vi "DAB Encode.vi"(10 "Message":string, 11 "image data":T1) -> (3 "Encoded Image":T1)   [LabVIEW 2020]
uses:
  <vilib>/picture/picture.llb/imagedata.ctl
panel:
  out "Encoded Bytes":i32
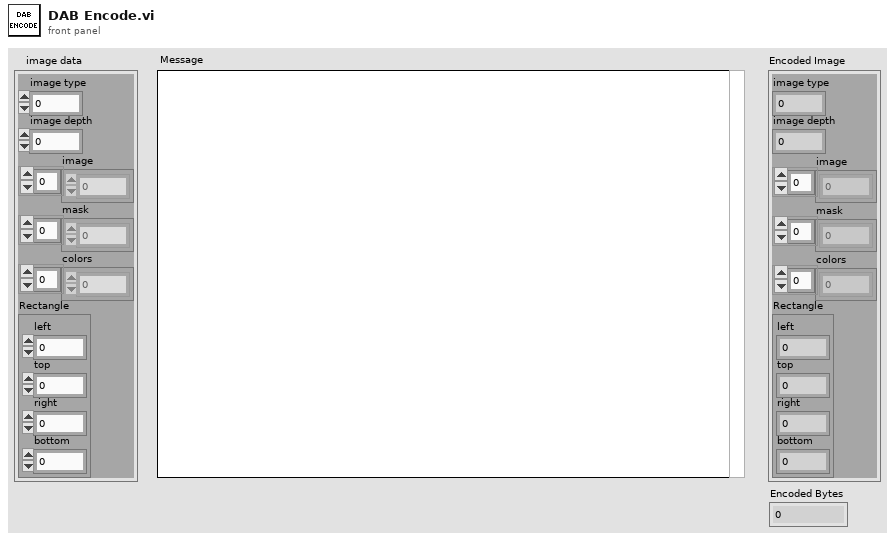
[diagram p1: front panel]
types:
  T1 = typedef "imagedata.ctl" = cluster{"image type":i32, "image depth":i32, "image":u8[], "mask":u8[], "colors":u32[], "Rectangle":cluster{"left":i16, "top":i16, "right":i16, "bottom":i16}}
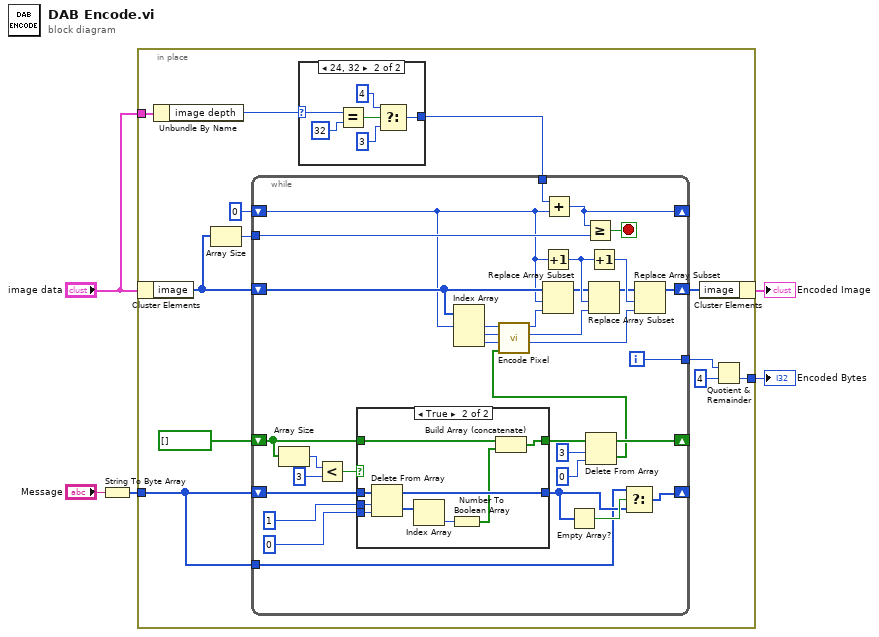
[diagram p0: block diagram]
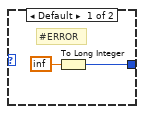
[diagram p3: hidden frame]
diagram:
  n1 = String To Byte Array(string="Message") -> (unsigned byte array=w2:u8[])
  n2 = in-place {
    in-place-border: "image data" -> [w17]
    in-place-border: w2 -> [w9]
    in-place-border: [w6] -> w1
    n3 = in-place-cluster #1("image data") -> ("image"=w13:u8[])
    n4 = Unbundle By Name(w17) -> ("image depth"=w16:i32)
    n5 = Array Size(array=w13) -> (size(s)=w12:i32)
    n6 = case shown="24, 32" w16 {
      selector: w16 -> [_ w70]
      tunnel: [w63 w65] -> w14
      frame Default {
        # "#ERROR"
        n7 = To Long Integer(number=inf) -> (32bit integer=w63:i32)
      }
      frame 24, 32 {
        n8 = Equal?(x=w70, y=32) -> (x = y?=w68:bool)
        n9 = Select(t=4, s=w68, f=3) -> (s? t:f=w65:i32)
      }
    }
    n10 = while {
      shift-right: [w35] -> w11
      shift-left: w13 -> [w44]
      shift-right: [w47] -> _
      shift-left: 0 -> [w43]
      tunnel: w14 -> [w51]
      tunnel: w12 -> [w46]
      shift-right: [w29] -> _
      shift-left: bool[] [] -> [w21]
      shift-right: [w24] -> _
      shift-left: w9 -> [w34]
      tunnel: w9 -> [w25]
      tunnel: [w23] -> w8
      i -> [w23]
      stop <- w45 stop-if-true
      n11 = Array Size(array=w21) -> (size(s)=w20:i32)
      n12 = Less?(x=w20, y=3) -> (x < y?=w18:bool)
      n13 = case shown="True" w18 {
        tunnel: w34 -> [w52 w62]
        tunnel: 0 ("index") -> [_ w61]
        tunnel: 1 ("length") -> [_ w60]
        tunnel: [w52 w59] -> w26
        tunnel: w21 -> [w53 w56]
        tunnel: [w53 w55] -> w31
        frame False {
        }
        frame True {
          n14 = Delete From Array(array=w62, length=w60, index=w61) -> (deleted portion=w58:u8[], array with subset deleted=w59:u8[])
          n15 = Index Array(array=w58) -> (element=w57:u8)  [unwired: 1 in]
          n16 = Number To Boolean Array(number=w57) -> (Boolean array=w54:bool[])
          n17 = Build Array (concatenate)(w56, w54) -> (w55:bool[])
        }
      }
      n18 = Index Array(array=w44, index #1=w43) -> (element #1=w50:u8, element #2=w49:u8, element #3=w48:u8)  [unwired: 2 in]
      n19 = Increment(x=w43) -> (x+1=w40:i32)
      n20 = Add(x=w51, y=w43) -> (x+y=w47:i32)
      n21 = Empty Array?(array=w26) -> (empty?=w27:bool)
      n22 = Greater Or Equal?(x=w47, y=w46) -> (x >= y?=w45:bool)
      n23 = Delete From Array(array=w31, length=3, index=0 ("length")) -> (deleted portion=w22:bool[], array with subset deleted=w29:bool[])
      n24 = call "Encode Pixel.vi"("3 Bits"=w22, "B"=w48, "G"=w49, "R"=w50) -> ("B 2"=w36:u8, "G 2"=w37:u8, "R 2"=w38:u8)  [unwired: 5 in]
      n25 = Replace Array Subset(array=w44, new element=w38, index=w43) -> (w39:u8[])
      n26 = Increment(x=w40) -> (x+1=w42:i32)
      n27 = Replace Array Subset(array=w39, new element=w37, index=w40) -> (w41:u8[])
      n28 = Select(t=w25, s=w27, f=w26) -> (s? t:f=w24:u8[])
      n29 = Replace Array Subset(array=w41, new element=w36, index=w42) -> (w35:u8[])
    }
    n30 = in-place-cluster #1("image"=w11) -> (→"Encoded Image":T1)
    n31 = Quotient & Remainder(x=w8, y=4) -> (floor(x/y)=w6:i32)  [unwired: 1 out]
  }
  "Encoded Bytes" <- w1
